vi "Open.vi"(5 "Dataset Variant":variant, 6 "Metadata":variant, 7 "Dataset[]":T1[](array[typedef]), 8 "error in (no error)":errorcluster, 9 "ScanSteps":i32, 10 "File":T2, 11 "CubeLogger in":refnum<class "CubeLogger.lvclass">) -> (0 "error out":errorcluster, 1 "Canceled?":bool, 2 "UUID[]":string[](array[string]), 3 "CubeLogger out":refnum<class "CubeLogger.lvclass">)   [LabVIEW 2018, in "CubeLogger.lvclass"]
uses:
  CubeLogger.lvclass
  File.ctl
  Dataset.ctl
  CubeLogger.lvclass/CubeLogger.ctl
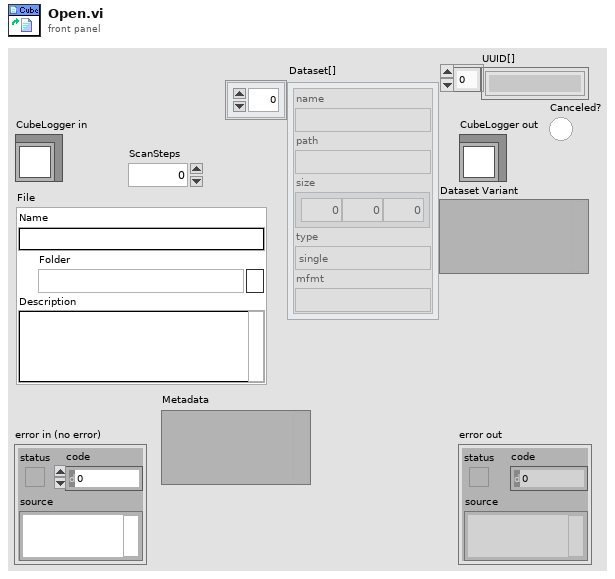
[diagram p1: front panel]
types:
  T1 = typedef "CubeLogger.lvclass/Dataset.ctl" = cluster{"name":string, "path":string, "size":i32[], "type":enum16{"single", "double", "uint8", "uint16", "uint32", "uint64", "int8", "int16", "int32", "int64"}, "mfmt":string}
  T2 = typedef "CubeLogger.lvclass/File.ctl" = cluster{"Name":string, "Folder":path, "Description":string}
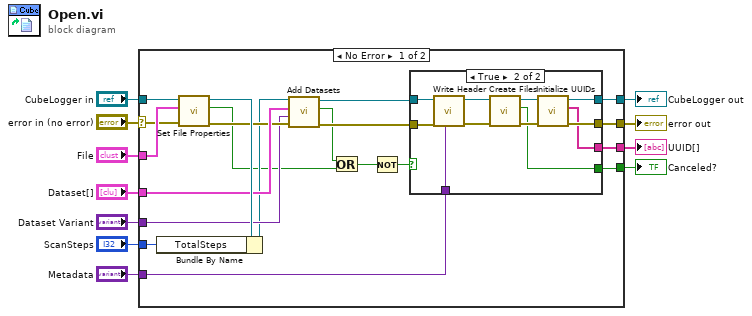
[diagram p0: block diagram]
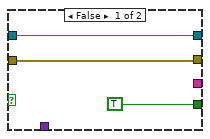
[diagram p2: hidden frame]
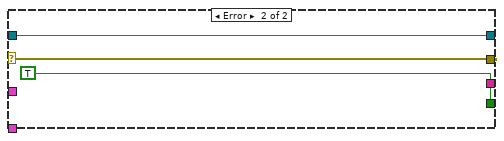
[diagram p3: hidden frame]
diagram:
  n1 = case shown="No Error" "error in (no error)" {
    selector: "error in (no error)" -> [w29 w48]
    tunnel: [w22 w48] -> w10
    tunnel: [w23 w47] -> w8
    tunnel: "CubeLogger in" -> [w31 w47]
    tunnel: "File" -> [w30 _]
    tunnel: "Dataset[]" -> [w27 _]
    tunnel: "Metadata" -> [w26 _]
    tunnel: "ScanSteps" -> [w18 _]
    tunnel: "Dataset Variant" -> [w24 _]
    tunnel: [w21 _] -> w2
    tunnel: [w12 TRUE] -> w1
    frame No Error {
      n2 = call "Set File Properties.vi"("error in (no error)"=w29, "File"=w30, "CubeLogger in"=w31) -> ("error out"=w25:errorcluster, "Canceled?"=w15:bool, "CubeLogger out"=w28:refnum<class "CubeLogger.lvclass">)  [unwired: 6 in]
      n3 = Bundle By Name(cluster=w28, "TotalSteps"=w18) -> (w19:refnum<class "CubeLogger.lvclass">)
      n4 = call-dynamic "Add Datasets.vi"("error in (no error)"=w25, "Dataset Variant"=w24, "Datasets"=w27, "CubeLogger in"=w19) -> ("error out"=w17:errorcluster, "Incomplete?"=w16:bool, "CubeLogger out"=w20:refnum<class "CubeLogger.lvclass">)  [unwired: 5 in]
      n5 = Or(x=w16, y=w15) -> (x .or. y?=w13:bool)
      n6 = Not(x=w13) -> (.not. x?=w14:bool)
      n7 = case shown="True" w14 {
        tunnel: w20 -> [w34 w37]
        tunnel: w26 -> [_ w35]
        tunnel: [w34 w45] -> w23
        tunnel: [w33 w44] -> w22
        tunnel: [_ w43] -> w21
        tunnel: w17 -> [w33 w36]
        tunnel: [TRUE w40] -> w12
        frame False {
        }
        frame True {
          n8 = call "Write Header.vi"("Metadata"=w35, "error in (no error)"=w36, "CubeLogger in"=w37) -> ("error out"=w38:errorcluster, "CubeLogger out"=w39:refnum<class "CubeLogger.lvclass">)  [unwired: 6 in, 1 out]
          n9 = call "Create Files.vi"("error in (no error)"=w38, "CubeLogger in"=w39) -> ("error out"=w41:errorcluster, "Canceled?"=w40:bool, "CubeLogger out"=w42:refnum<class "CubeLogger.lvclass">)  [unwired: 7 in]
          n10 = call "Initialize UUIDs.vi"("error in (no error)"=w41, "CubeLogger in"=w42) -> ("error out"=w44:errorcluster, "UUID[]"=w43:string[], "CubeLogger out"=w45:refnum<class "CubeLogger.lvclass">)  [unwired: 7 in]
        }
      }
    }
    frame Error {
    }
  }
  "error out" <- w10
  "CubeLogger out" <- w8
  "UUID[]" <- w2
  "Canceled?" <- w1
